vi "WPI_ERRMotorControlCANJaguarDevice.vi"(7 "Device Number":u8) -> (8 "error out":errorcluster)   [LabVIEW 2017]
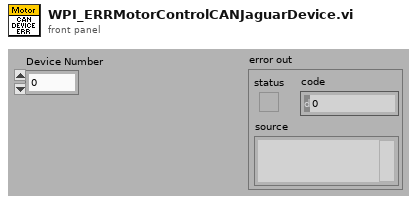
[diagram p1: front panel]
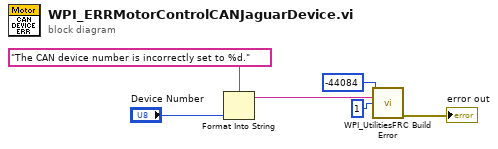
[diagram p0: block diagram]
diagram:
  n1 = Format Into String(format string="The CAN device number is incorrectly set to %d.", "Device Number") -> (resulting string=w1:string)  [unwired: 2 in, 1 out]
  n2 = call <vilib>:"WPI_UtilitiesFRC Build Error.vi"("error code"=-44084 ("code"), "extra error text"=w1, "chain levels to remove (1)"=1) -> ("error out"=→"error out":errorcluster)  [unwired: 2 in, 10 out]
